vi "loadAndFormatValues.vi"(5 "error in (no error)":errorcluster, 7 "configuration":T2, 9 "channel names":string[](array[string]), 10 "group names":string[](array[string]), 11 "TDMS descriptor array":T1(array[cluster])) -> (0 "error out":errorcluster, 1 "graph y names":string, 2 "graph x names":string, 3 "TDMS descriptor array out":T1(array[cluster]), 4 "waveform values":waveform(dbl)[](array[waveform]), 6 "table values":string[][](array[string]), 8 "table headers":string[](array[string]))   [LabVIEW 2015]
uses:
  <vilib>/Utility/tdmsutil.llb/fileViewerConfigData.ctl
panel:
  out "tdms file out":refnum<k34>
  in  "tdms file":refnum<k34>
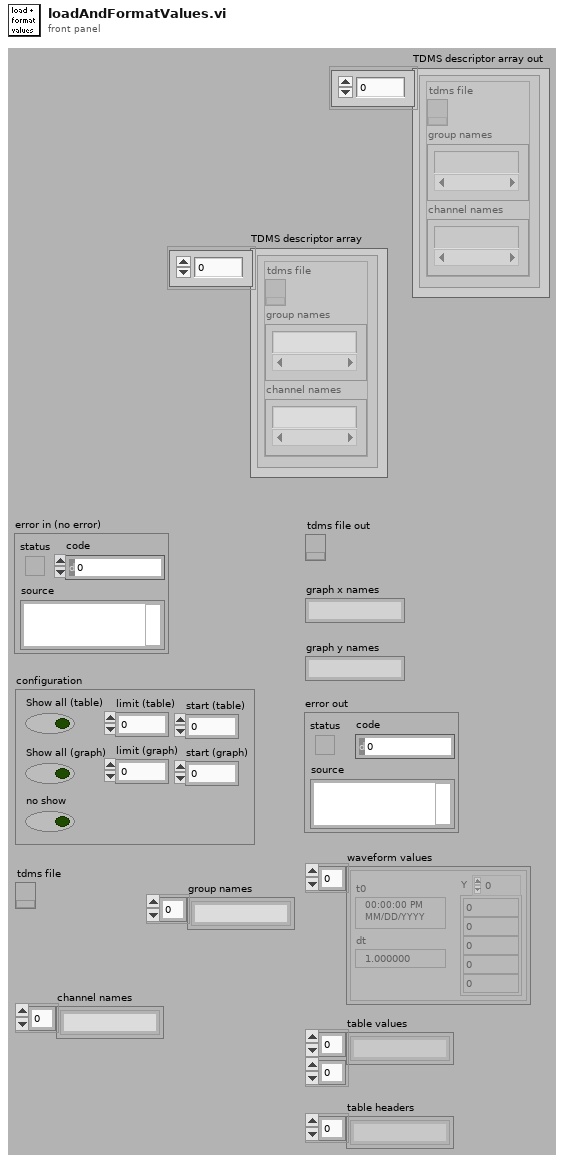
[diagram p1: front panel]
types:
  T1 = cluster{"tdms file ":refnum<k34>, "group names":string[], "channel names":string[]}[]
  T2 = typedef "fileViewerConfigData.ctl" = cluster{"Show all (table)":bool, "Show all (graph)":bool, "limit (table)":u64, "limit (graph)":u64, "no show":bool, "start (table)":u64, "start (graph)":u64}
  T3 = cluster{"tdms file ":refnum<k34>, "group names":string[], "channel names":string[]}
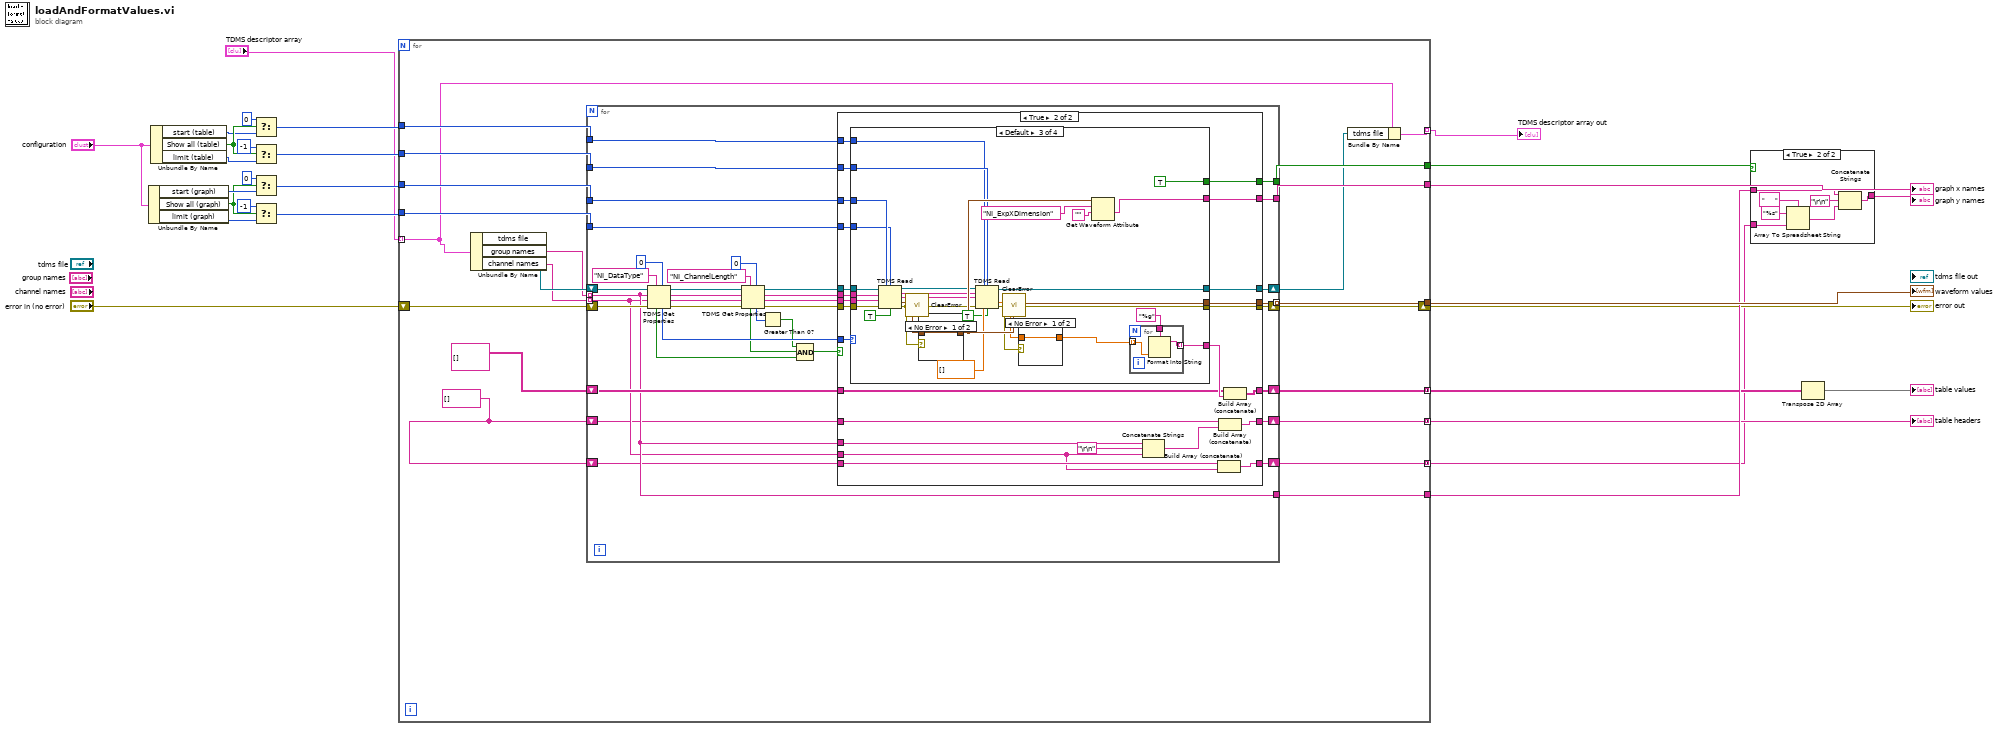
[diagram p0: block diagram]
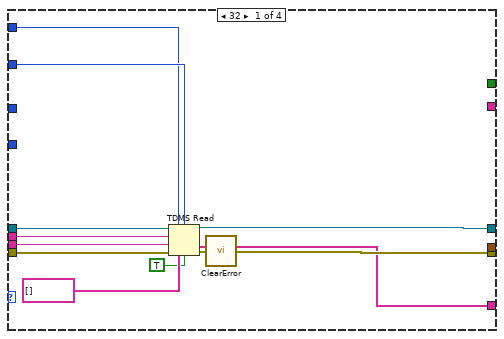
[diagram p3: hidden frame]
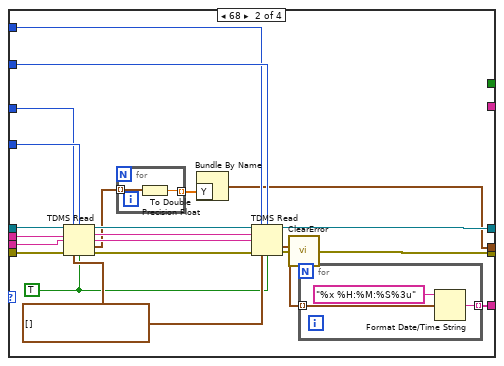
[diagram p4: hidden frame]
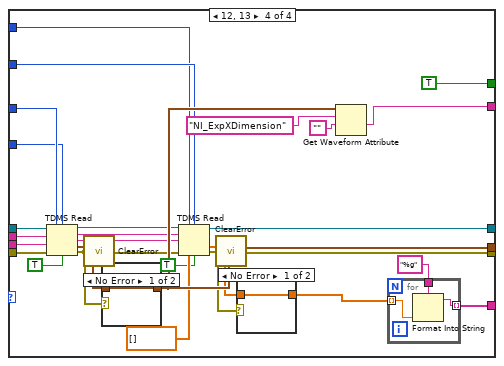
[diagram p7: hidden frame]
diagram:
  n1 = Unbundle By Name("configuration") -> ("start (graph)"=w23:u64, "Show all (graph)"=w22:bool, "limit (graph)"=w21:u64)
  n2 = Unbundle By Name("configuration") -> ("start (table)"=w16:u64, "Show all (table)"=w17:bool, "limit (table)"=w18:u64)
  n3 = Select(t=u64 0, s=w17, f=w16) -> (s? t:f=w19:u64)
  n4 = Select(t=i64 -1 ("count (-1: all)"), s=w17, f=w18) -> (s? t:f=w20:u64)
  n5 = Select(t=u64 0, s=w22, f=w23) -> (s? t:f=w27:u64)
  n6 = Select(t=i64 -1 ("count (-1: all)"), s=w22, f=w21) -> (s? t:f=w26:u64)
  n7 = for {
    tunnel: w27 -> [w49]
    tunnel: w26 -> [w48]
    tunnel: w20 -> [w47]
    tunnel: w19 -> [w46]
    tunnel: [w44] -> w12
    tunnel: [w43] -> w11
    tunnel: [w42] -> w10
    tunnel: [w41] -> w8
    tunnel: [w39] -> w5 mode=concatenating
    tunnel: [w38] -> w4 mode=concatenating
    tunnel: [w37] -> w3 mode=concatenating
    shift-right: [w40] -> w7
    shift-left: "error in (no error)" -> [w45]
    tunnel: "TDMS descriptor array" -> [w33] mode=indexing
    tunnel: [w31] -> w1 mode=indexing
    w29 = string[] []
    n8 = Unbundle By Name(w33) -> ("tdms file"=w36:refnum<k34>, "group names"=w35:string[], "channel names"=w34:string[])
    n9 = for {
      tunnel: w49 -> [w85]
      tunnel: w48 -> [w84]
      tunnel: [w82] -> w44 mode=indexing
      tunnel: w34 -> [w54] mode=indexing
      shift-right: [w83] -> w40
      shift-left: w45 -> [w80]
      shift-right: [w86] -> w32
      shift-left: w36 -> [w79]
      tunnel: w35 -> [w55] mode=indexing
      tunnel: [w81] -> w42
      tunnel: [w55] -> w41
      tunnel: [w75] -> w43
      tunnel: w47 -> [w74]
      tunnel: w46 -> [w73]
      shift-right: [w56] -> w39
      shift-left: string[][] [] -> [w57]
      shift-right: [w52] -> w38
      shift-left: w29 -> [w53]
      shift-right: [w50] -> w37
      shift-left: w29 -> [w51]
      n10 = TDMS Get Properties(5:u16 0, 7:"NI_DataType" ("property name"), 8:w80, 9:w54, 10:w55, 11:w79) -> (0:w72:errorcluster, 1:w65:string, 2:w66:string, 3:w71:refnum<k34>, 4:w76:u16, 6:w59:bool)
      n11 = TDMS Get Properties(5:u64 0, 7:"NI_ChannelLength" ("property name"), 8:w72, 9:w65, 10:w66, 11:w71) -> (0:w70:errorcluster, 1:w69:string, 2:w68:string, 3:w67:refnum<k34>, 4:w62:u64, 6:w60:bool)
      n12 = Greater Than 0?(x=w62) -> (x > 0?=w61:bool)
      n13 = Compound Arithmetic op=AND(w61, w60, w59) -> (w58:bool)
      n14 = case shown="True" w58 {
        tunnel: [w91 w116] -> w86
        tunnel: w85 -> [_ w115]
        tunnel: w84 -> [_ w114]
        tunnel: [w90 w104] -> w83
        tunnel: [_ w103] -> w82
        tunnel: [_ w113] -> w81
        tunnel: w67 -> [w91 w112]
        tunnel: w70 -> [w90 w111]
        tunnel: w68 -> [_ w110]
        tunnel: w69 -> [_ w109]
        tunnel: w76 -> [_ w108]
        tunnel: [_ w107] -> w75
        tunnel: w74 -> [_ w106]
        tunnel: w73 -> [_ w105]
        tunnel: w57 -> [w89 w100]
        tunnel: [w89 w101] -> w56
        tunnel: w55 -> [_ w98]
        tunnel: w54 -> [_ w93]
        tunnel: w53 -> [w88 w97]
        tunnel: [w88 w95] -> w52
        tunnel: w51 -> [w87 w94]
        tunnel: [w87 w92] -> w50
        frame False {
        }
        frame True {
          n15 = case shown="Default" w108 {
            tunnel: [w122 w149 w166 w200] -> w116
            tunnel: w115 -> [_ w133 w184 w218]
            tunnel: w114 -> [_ w134 w183 w217]
            tunnel: [w123 w150 w167 w201] -> w104
            tunnel: [w121 w148 w159 w193] -> w102
            tunnel: [_ w130 w174 w208] -> w103
            tunnel: [_ _ w156 w190] -> w113
            tunnel: w112 -> [w128 w142 w180 w214]
            tunnel: w111 -> [w125 w143 w179 w213]
            tunnel: w110 -> [w127 w141 w178 w212]
            tunnel: w109 -> [w126 w140 w177 w211]
            tunnel: [_ _ TRUE TRUE] -> w107
            tunnel: w106 -> [w120 w146 w165 w199]
            tunnel: w105 -> [w119 w145 w164 w198]
            frame 32 {
              n16 = TDMS Read(0:w128, 1:w119, 2:w120, 5:w127, 7:w126, 11:w125, 12:string[] [], 13:TRUE ("return channels in file order? (F)")) -> (4:w122:refnum<k34>, 10:w121:string[], 15:w118:errorcluster)  [unwired: 3 out]
              n17 = call <vilib>:"ClearError.vi"("error in (no error)"=w118) -> ("error out"=w123:errorcluster)
            }
            frame 68 {
              w135 = TRUE ("return channels in file order? (F)")
              w136 = timestamp[] []
              n18 = TDMS Read(0:w142, 1:w133, 2:w134, 5:w141, 7:w140, 11:w143, 12:w136, 13:w135) -> (4:w137:refnum<k34>, 6:w138:string, 8:w139:string, 10:w132:timestamp[], 15:w129:errorcluster)  [unwired: 1 out]
              n19 = for {
                tunnel: w132 -> [w152] mode=indexing
                tunnel: [w151] -> w131 mode=indexing
                n20 = To Double Precision Float(number=w152) -> (double precision float=w151:dbl)
              }
              n21 = Bundle By Name("Y"=w131) -> (w130:waveform(dbl))  [unwired: 1 in]
              n22 = TDMS Read(0:w137, 1:w145, 2:w146, 5:w138, 7:w139, 11:w129, 12:w136, 13:w135) -> (4:w149:refnum<k34>, 10:w147:timestamp[], 15:w144:errorcluster)  [unwired: 3 out]
              n23 = call <vilib>:"ClearError.vi"("error in (no error)"=w144) -> ("error out"=w150:errorcluster)
              n24 = for {
                tunnel: [w155] -> w148 mode=indexing
                tunnel: w147 -> [w154] mode=indexing
                n25 = Format Date/Time String(time format string (%c)="%x %H:%M:%S%3u", seconds (now)=w154) -> (date/time string=w155:string)  [unwired: 1 in]
              }
            }
            frame Default {
              n26 = TDMS Read(0:w180, 1:w184, 2:w183, 5:w178, 7:w177, 11:w179, 13:TRUE ("return channels in file order? (F)")) -> (4:w173:refnum<k34>, 6:w171:string, 8:w170:string, 10:w175:waveform(dbl), 15:w162:errorcluster)  [unwired: 1 in, 1 out]
              n27 = call <vilib>:"ClearError.vi"("error in (no error)"=w162) -> ("error out"=w172:errorcluster)
              n28 = case shown="No Error" w172 {
                tunnel: w175 -> [w189 _]
                tunnel: [w189 _] -> w174
                frame No Error {
                }
                frame Error {
                }
              }
              n29 = TDMS Read(0:w173, 1:w164, 2:w165, 5:w171, 7:w170, 11:w172, 12:dbl[] [], 13:TRUE ("return channels in file order? (F)")) -> (4:w166:refnum<k34>, 10:w169:dbl[], 15:w163:errorcluster)  [unwired: 3 out]
              n30 = call <vilib>:"ClearError.vi"("error in (no error)"=w163) -> ("error out"=w167:errorcluster)
              n31 = case shown="No Error" w167 {
                tunnel: w169 -> [w188 _]
                tunnel: [w188 _] -> w160
                frame No Error {
                }
                frame Error {
                }
              }
              n32 = Get Waveform Attribute(5:"", 6:"NI_ExpXDimension" ("name"), 7:w174) -> (1:w156:string)  [unwired: 1 in, 3 out]
              n33 = for {
                tunnel: "%g" ("format string") -> [w187]
                tunnel: w160 -> [w186] mode=indexing
                tunnel: [w185] -> w159 mode=indexing
                n34 = Format Into String(format string=w187, w186) -> (resulting string=w185:string)  [unwired: 2 in, 1 out]
              }
            }
            frame 12, 13 {
              n35 = TDMS Read(0:w214, 1:w218, 2:w217, 5:w212, 7:w211, 11:w213, 13:TRUE ("return channels in file order? (F)")) -> (4:w207:refnum<k34>, 6:w205:string, 8:w204:string, 10:w209:waveform(dbl), 15:w196:errorcluster)  [unwired: 1 in, 1 out]
              n36 = call <vilib>:"ClearError.vi"("error in (no error)"=w196) -> ("error out"=w206:errorcluster)
              n37 = case shown="No Error" w206 {
                tunnel: w209 -> [w223 _]
                tunnel: [w223 _] -> w208
                frame No Error {
                }
                frame Error {
                }
              }
              n38 = TDMS Read(0:w207, 1:w198, 2:w199, 5:w205, 7:w204, 11:w206, 12:cdb[] [], 13:TRUE ("return channels in file order? (F)")) -> (4:w200:refnum<k34>, 10:w203:cdb[], 15:w197:errorcluster)  [unwired: 3 out]
              n39 = call <vilib>:"ClearError.vi"("error in (no error)"=w197) -> ("error out"=w201:errorcluster)
              n40 = case shown="No Error" w201 {
                tunnel: w203 -> [w222 _]
                tunnel: [w222 _] -> w194
                frame No Error {
                }
                frame Error {
                }
              }
              n41 = Get Waveform Attribute(5:"", 6:"NI_ExpXDimension" ("name"), 7:w208) -> (1:w190:string)  [unwired: 1 in, 3 out]
              n42 = for {
                tunnel: "%g" ("format string") -> [w221]
                tunnel: w194 -> [w220] mode=indexing
                tunnel: [w219] -> w193 mode=indexing
                n43 = Format Into String(format string=w221, w220) -> (resulting string=w219:string)  [unwired: 2 in, 1 out]
              }
            }
          }
          n44 = Concatenate Strings(w98, "\r\n", w93) -> (w96:string)
          n45 = Build Array (concatenate)(w94, w93) -> (w92:string[])
          n46 = Build Array (concatenate)(w97, w96) -> (w95:string[])
          n47 = Build Array (concatenate)(w100, w102) -> (w101:string[][])
        }
      }
    }
    n48 = Bundle By Name(cluster=w33, "tdms file"=w32) -> (w31:T3)
  }
  "waveform values" <- w12
  "graph x names" <- w10
  "table headers" <- w4
  "error out" <- w7
  "TDMS descriptor array out" <- w1
  n49 = case shown="True" w11 {
    tunnel: w3 -> [_ w229]
    tunnel: w8 -> [_ w226]
    tunnel: [_ w225] -> w9
    frame False {
    }
    frame True {
      n50 = Array To Spreadsheet String(delimiter (Tab)="     ", array=w229, 3:"%s" ("format string")) -> (spreadsheet string=w227:string)
      n51 = Concatenate Strings(w226, "\r\n", w227) -> (w225:string)
    }
  }
  "graph y names" <- w9
  n52 = Transpose 2D Array(2D array=w5) -> (transposed array=→"table values":string[][])
